vi "Draw.vi"(8 "error in (no error)":errorcluster, 11 "Snake in":refnum<class "SnakeGame.lvclass">) -> (0 "error out":errorcluster, 3 "Snake out":refnum<class "SnakeGame.lvclass">)   [LabVIEW 2019, in "RT_Game.lvlib" / "SnakeGame.lvclass"]
uses:
  SnakeGame.lvclass
  C:/Users/FreshBob/Dropbox/VIs/myRIO_GameConsole/RT/RT_Game/Game/Game.lvclass
  SnakeGame.lvclass/SnakeGame.ctl
  Game/Game.lvclass
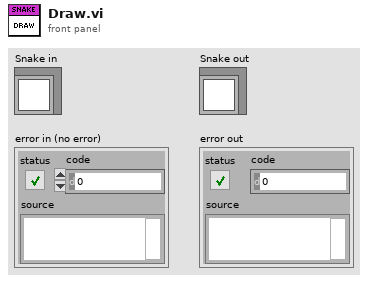
[diagram p1: front panel]
types:
  T1 = typedef "RT_Game.lvlib/Game.lvclass/Coordinate.ctl" = cluster{"x":i16, "y":i16}
  T2 = typedef "RT_Game.lvlib/SnakeGame.lvclass/SnakeData.ctl" = cluster{"Length":i16, "Direction":T3, "Position":T1, "Coordinates":T4[], "ScorePosition":T1, "Dead?":bool, "Color":fxp<+,3,3>, "LastDirection":T3}
  T3 = typedef "RT_Game.lvlib/SnakeGame.lvclass/Direction.ctl" = enum16{"Up", "Left", "Down", "Right"}
  T4 = typedef "RT_Game.lvlib/SnakeGame.lvclass/CoordinateData.ctl" = cluster{"Coordinate":T1, "TileCode":string}
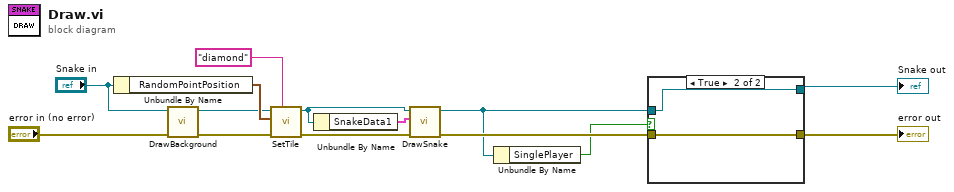
[diagram p0: block diagram]
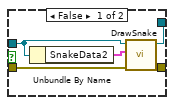
[diagram p2: hidden frame]
diagram:
  n1 = Unbundle By Name("Snake in") -> ("RandomPointPosition"=w12:T1)
  n2 = call "DrawBackground.vi"("error in (no error)"="error in (no error)", "Snake in"="Snake in") -> ("error out"=w7:errorcluster, "Snake out"=w9:refnum<class "SnakeGame.lvclass">)  [unwired: 8 in]
  n3 = call "SetTile.vi"("TileCode"="diamond", "error in (no error)"=w7, "Coordinates"=w12, "Game in"=w9) -> ("error out"=w11:errorcluster, "Game out"=w6:refnum<class "SnakeGame.lvclass">)  [unwired: 6 in]
  n4 = Unbundle By Name(w6) -> ("SnakeData1"=w3:T2)
  n5 = call "DrawSnake.vi"("error in (no error)"=w11, "SnakeData"=w3, "Snake in"=w6) -> ("error out"=w14:errorcluster, "Snake out"=w2:refnum<class "SnakeGame.lvclass">)  [unwired: 7 in]
  n6 = Unbundle By Name(w2) -> ("SinglePlayer"=w1:bool)
  n7 = case shown="True" w1 {
    tunnel: w14 -> [w19 w20]
    tunnel: w2 -> [w18 w21]
    tunnel: [w17 w21] -> w5
    tunnel: [w16 w20] -> w4
    frame False {
      n8 = Unbundle By Name(w18) -> ("SnakeData2"=w15:T2)
      n9 = call "DrawSnake.vi"("error in (no error)"=w19, "SnakeData"=w15, "Snake in"=w18) -> ("error out"=w16:errorcluster, "Snake out"=w17:refnum<class "SnakeGame.lvclass">)  [unwired: 7 in]
    }
    frame True {
    }
  }
  "Snake out" <- w5
  "error out" <- w4
